vi "Error Message.vi"(8 "error in (no error)":errorcluster, 10 "Error Code in":u16, 11 "VISA resource name":refnum<visa-resource-name>) -> (0 "error out":errorcluster, 1 "Error Message":string, 3 "VISA resource name out":refnum<visa-resource-name>)   [LabVIEW 2017, in "Temptronic TP04300.lvlib"]
uses:
  Temptronic TP04300.lvlib
  TP04300 EROR.ctl
  TP04300 EROR 4000 Compatible.ctl
  4000 Compatible.vi
panel:
  out "TP04300 EROR 4000 Compatible":T1
  out "TP04300 EROR":T2
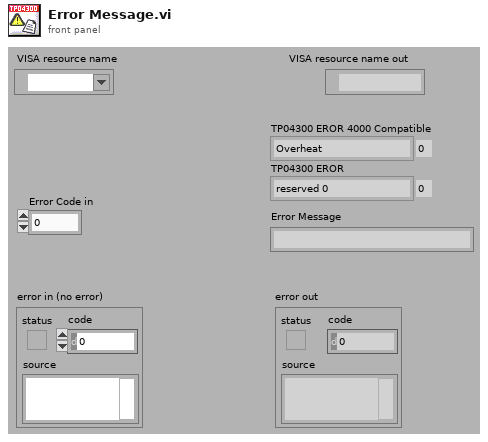
[diagram p1: front panel]
types:
  T1 = typedef "Temptronic TP04300.lvlib/TP04300 EROR 4000 Compatible.ctl" = enum16{"Overheat", "Air Open Loop", "Setpoint out of Range", "Low Flow", "Low Pressure", "No Purge Flow", "Open Purge Temperature Sensor", "Internal Error", "DUT Open Loop Failure", "Flow Sensor Failure", "Purge Heat Failure", "reserved 11", "reserved 12", "Improper Software", "No DUT Sensor Selected", "reserved 15"}
  T2 = typedef "Temptronic TP04300.lvlib/TP04300 EROR.ctl" = enum16{"reserved 0", "reserved 1", "reserved 2", "Controller Failure", "AC Absent", "Air Open Loop", "Low Temperature Limit", "High Temperature Limit", "Main TC Failure", "Low Pressure", "Low Flow Limit", "Air Flow Open Loop", "DUT Sensor Failure", "reserved 14", "reserved 15"}
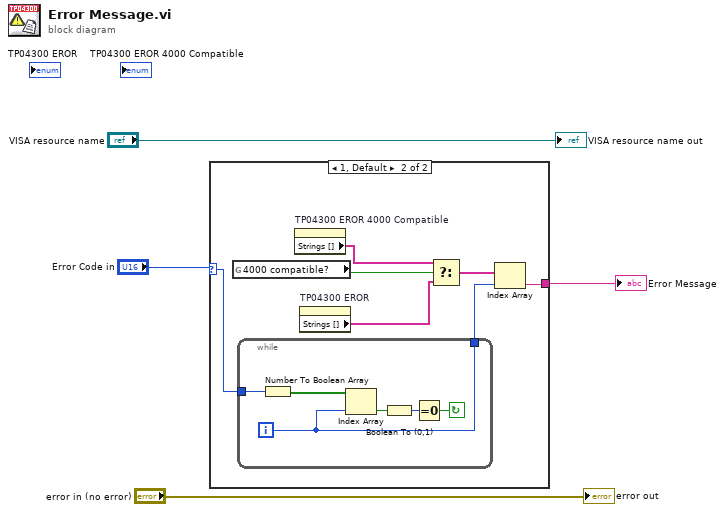
[diagram p0: block diagram]
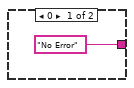
[diagram p2: hidden frame]
diagram:
  n1 = case shown="1, Default" "Error Code in" {
    selector: "Error Code in" -> [_ w7]
    tunnel: ["No Error" w8] -> w2
    frame 0 {
    }
    frame 1, Default {
      n2 = global read "4000 Compatible.vi" "4000 compatible?"() -> (w9:bool)
      n3 = while {
        tunnel: w7 -> [w18]
        tunnel: [w13] -> w6
        i -> [w13]
        stop <- w14 continue-if-true
        n4 = Number To Boolean Array(number=w18) -> (Boolean array=w17:bool[])
        n5 = Index Array(array=w17, index=w13) -> (element=w16:bool)
        n6 = Boolean To (0,1)(Boolean=w16) -> (0, 1=w15:i16)
        n7 = Equal To 0?(x=w15) -> (x = 0?=w14:bool)
      }
      n8 = property on="TP04300 EROR 4000 Compatible" class="Enum (strict)"() -> ("Strings []"=w12:string[])  [unwired: 2 in, 2 out]
      n9 = property on="TP04300 EROR" class="Enum (strict)"() -> ("Strings []"=w11:string[])  [unwired: 2 in, 2 out]
      n10 = Select(t=w12, s=w9, f=w11) -> (s? t:f=w10:string[])
      n11 = Index Array(array=w10, index=w6) -> (element=w8:string)
    }
  }
  "Error Message" <- w2
  "error out" <- "error in (no error)"
  "VISA resource name out" <- "VISA resource name"
